vi "SQUARE WITH SIGN.vi"(1 "Input":dbl) -> (0 "Output":dbl)   [LabVIEW 2015]
doc: "Squaring an input provides higher precision with small values without sacrificing maximum speed (i.e. 1 becomes 1, 0.75 becomes 0.56, 0.5 becomes 0.25, ete). However, squaring values also has the effect of applying an absolute value function to an input. This convenience method allows you to square an input without making negative values positive."
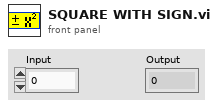
[diagram p1: front panel]
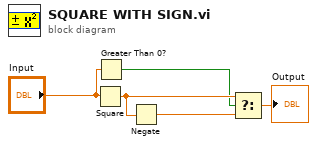
[diagram p0: block diagram]
diagram:
  n1 = Square(x="Input") -> (x^2=w4:dbl)
  n2 = Greater Than 0?(x="Input") -> (x > 0?=w2:bool)
  n3 = Negate(x=w4) -> (-x=w3:dbl)
  n4 = Select(t=w4, s=w2, f=w3) -> (s? t:f=→"Output":dbl)
